vi "Read Color Pair.vi"(8 "error in (no error)":errorcluster, 9 "Active Plot":i32, 11 "3D Pie in":refnum<class "3D Pie.lvclass">) -> (0 "error out":errorcluster, 2 "Color Pair Array":cluster{"Color":u32, "String":string}[](array[cluster]), 3 "3D Pie out":refnum<class "3D Pie.lvclass">)   [LabVIEW 2017, in "3D Pie.lvclass"]
uses:
  <vilib>/Math Plots/3D Math Plots/3D Pie/3D Pie/3D Pie.lvclass
  <vilib>/Math Plots/3D Math Plots/3D Pie/3D Pie/3D Pie.lvclass/3D Pie.ctl
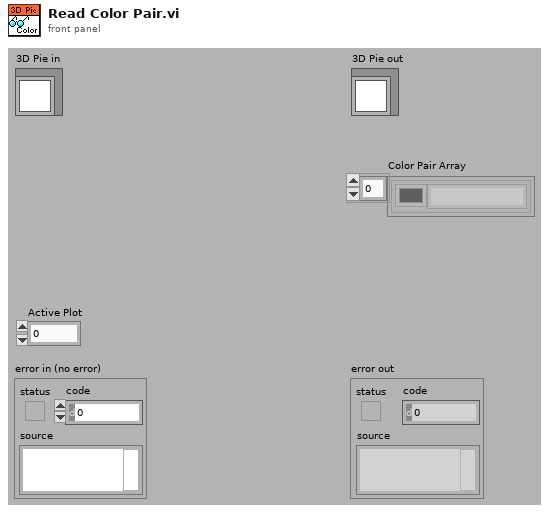
[diagram p1: front panel]
types:
  T1 = typedef "3D Pie.lvclass/3D Pie Property Array.ctl" = T2[]
  T2 = typedef "3D Pie.lvclass/3D Pie Property.ctl" = cluster{"General Property":cluster{"Plot Name":string, "Coordinate System":enum16{"Cartesian", "Cylindrical", "Spherical"}, "Opacity":sgl}, "Projection Property":cluster{"Draw XY":bool, "Draw YZ":bool, "Draw XZ":bool}, "Plot Property":cluster{"Line Style":T3, "Line Width":sgl, "Line Color":u32, "Antialiasing":bool}, "Pie Property":cluster{"Pie Height":sgl, "Pie Center":cluster{"X":sgl, "Y":sgl, "Z":sgl}, "Label Mode":enum16{"None", "Show Percentage", "Show String"}, "Label Size":u16, "Label Color":u32, "Color Pair Array":cluster{"Color":u32, "String":string}[], "Slice Offset?":bool}}
  T3 = typedef "3D Plot.lvclass/Line Type.ctl" = enum16{"None", "Solid", "Dash", "Dot", "Dash Dot"}
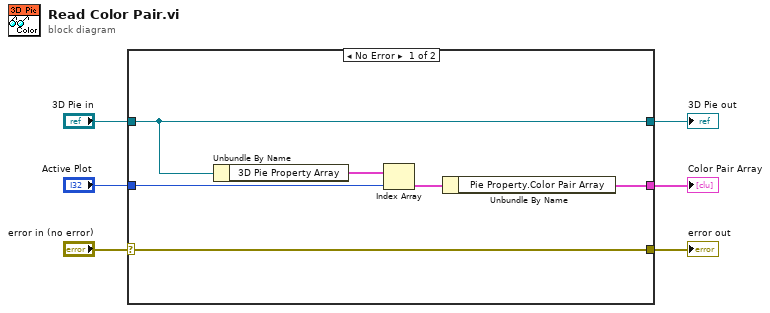
[diagram p0: block diagram]
diagram:
  n1 = case shown="No Error" "error in (no error)" {
    selector: "error in (no error)" -> [w12 w14]
    tunnel: "3D Pie in" -> [w11 w13]
    tunnel: [w11 w13] -> w3
    tunnel: [w12 w14] -> w2
    tunnel: "Active Plot" -> [w9 _]
    tunnel: [w7 _] -> w4
    frame No Error {
      n2 = Unbundle By Name(w11) -> ("3D Pie Property Array"=w10:T1)
      n3 = Index Array(array=w10, index=w9) -> (element=w8:T2)
      n4 = Unbundle By Name(w8) -> ("Pie Property.Color Pair Array"=w7:cluster{"Color":u32, "String":string}[])
    }
    frame Error {
    }
  }
  "error out" <- w2
  "3D Pie out" <- w3
  "Color Pair Array" <- w4
